vi "CloseFile.vi"(7 "Independent?":bool, 8 "error in (no error)":errorcluster, 10 "notifier in":refnum<notifier>, 11 "Refnum in":refnum<k34>) -> (0 "error out":errorcluster, 1 "Notifier out":refnum<notifier>, 2 "Not a refnum out":refnum<k34>, 3 "File Close action out":enum16{"Prompt", "Keep", "Archive", "Trash"}(ring))   [LabVIEW 2018]
panel:
  # "warning this VI is cloned when opened to prevent notification isses when called simultaneously make sure to edit the VI opened from explorer."
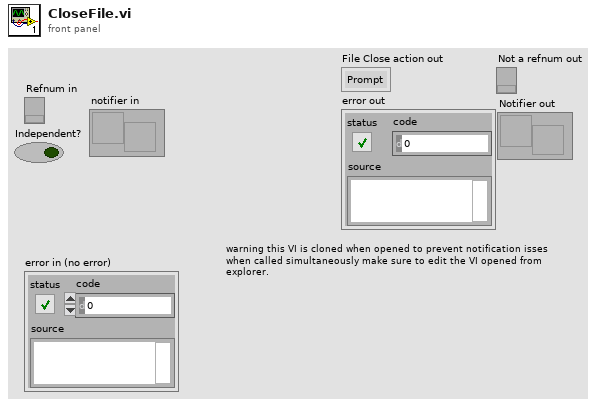
[diagram p1: front panel]
types:
  T1 = enum16{"Left Button", "Center Button", "Right Button", "Window Close"}
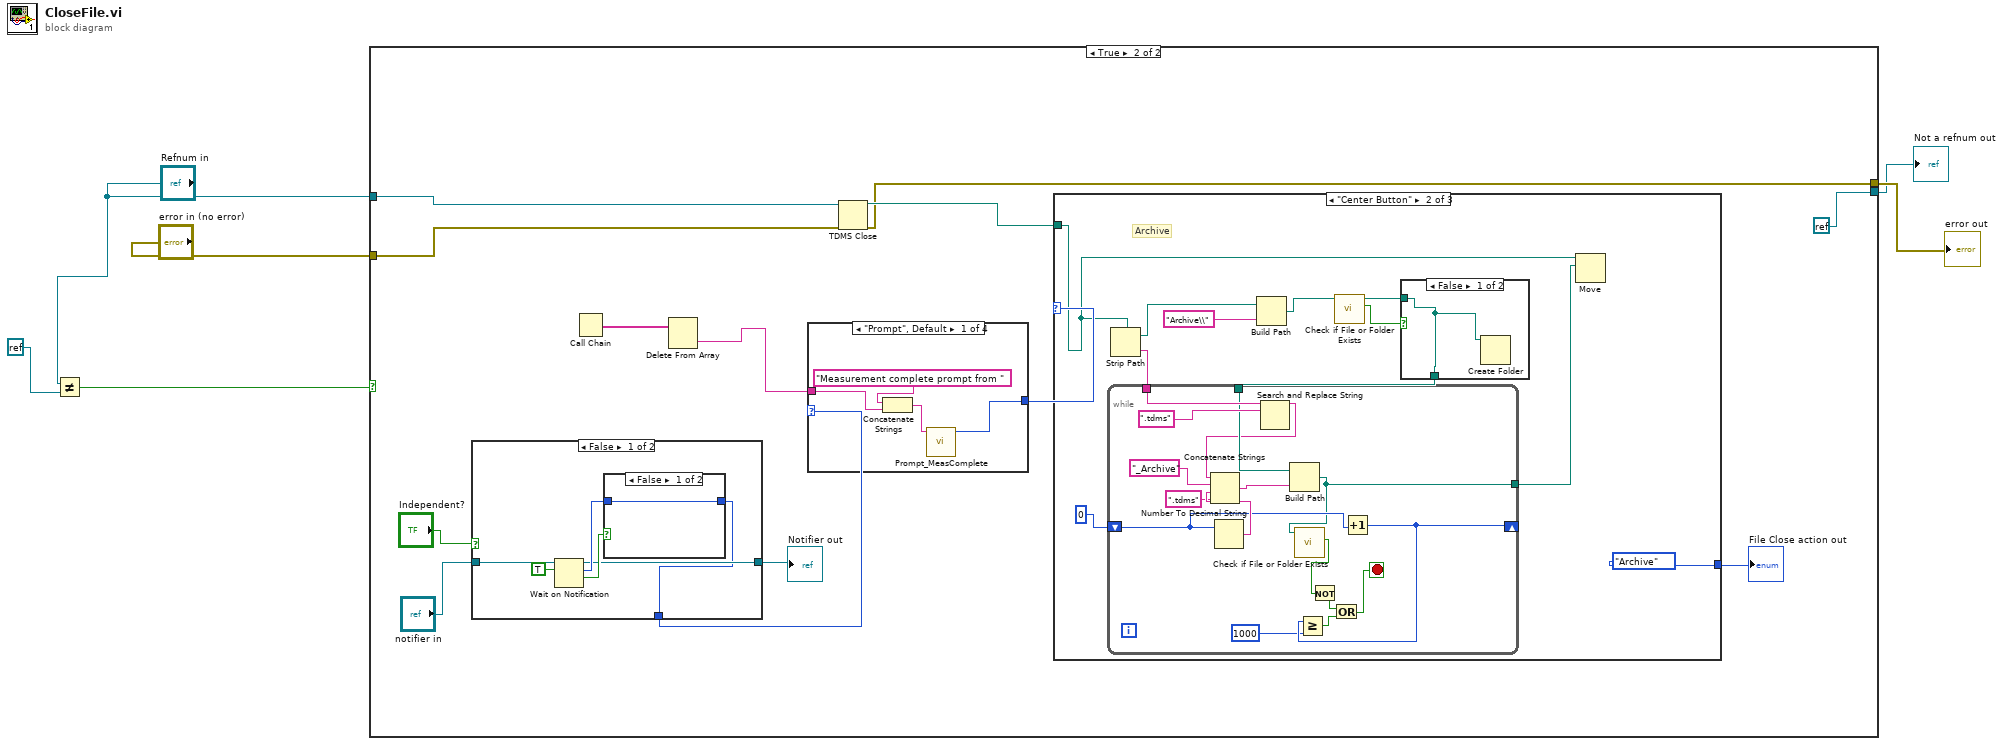
[diagram p0: block diagram]
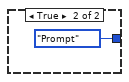
[diagram p3: hidden frame]
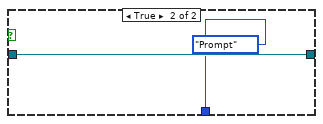
[diagram p4: hidden frame]
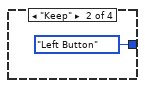
[diagram p5: hidden frame]
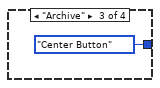
[diagram p6: hidden frame]
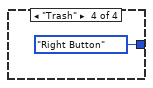
[diagram p7: hidden frame]
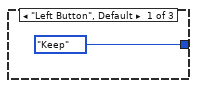
[diagram p8: hidden frame]
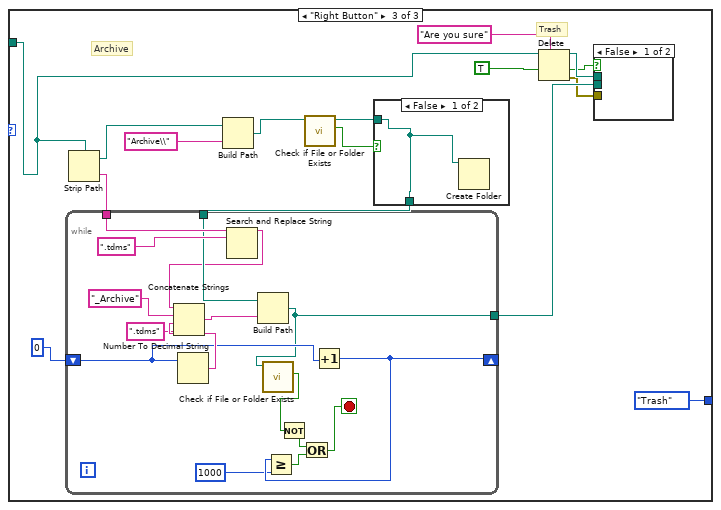
[diagram p10: hidden frame]
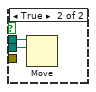
[diagram p11: hidden frame]
diagram:
  n1 = Not Equal?(x="Refnum in", y=refnum<k0> refnum) -> (x != y?=w3:bool)
  n2 = case shown="True" w3 {
    tunnel: "error in (no error)" -> [w7 w20]
    tunnel: "Refnum in" -> [w8 w18]
    tunnel: [w8 refnum<k0> refnum] -> w1
    tunnel: [w7 w16] -> w2
    frame False {
    }
    frame True {
      n3 = case shown="False" "Independent?" {
        tunnel: "notifier in" -> [w27 w31]
        tunnel: [w24 w31] -> w14
        tunnel: [w23 enum16{"Prompt", "Keep", "Archive", "Trash"}."Prompt" ("Action")] -> w11
        frame False {
          n4 = Wait on Notification(notifier=w27, ignore previous (F)=TRUE) -> (notifier out=w24:refnum<notifier>, notification=w25:enum16{"Prompt", "Keep", "Archive", "Trash"}, timed out?=w26:bool)  [unwired: 2 in, 1 out]
          n5 = case shown="False" w26 {
            tunnel: w25 -> [w28 _]
            tunnel: [w28 enum16{"Prompt", "Keep", "Archive", "Trash"}."Prompt" ("Action")] -> w23
            frame False {
            }
            frame True {
            }
          }
        }
        frame True {
        }
      }
      "Notifier out" <- w14
      n6 = Call Chain() -> (call chain=w10:string[])
      n7 = Delete From Array "Delete From Array"(array=w10) -> (deleted portion=w9:string)  [unwired: 2 in, 1 out]
      n8 = case shown="\"Prompt\", Default" w11 {
        tunnel: [w35 T1."Left Button" ("Which Button?") T1."Center Button" ("Which Button?") T1."Right Button" ("Which Button?")] -> w19
        tunnel: w9 -> [w34 _ _ _]
        frame "Prompt", Default {
          n9 = Concatenate Strings("Measurement complete prompt from " ("message"), w34) -> (w32:string)
          n10 = call "Prompt_MeasComplete.vi"("message"=w32) -> ("Which Button?"=w35:T1)  [unwired: 10 in]
        }
        frame "Keep" {
        }
        frame "Archive" {
        }
        frame "Trash" {
        }
      }
      n11 = TDMS Close(8:w20, 11:w18) -> (0:w16:errorcluster, 3:w21:path)
      n12 = case shown="\"Center Button\"" w19 {
        tunnel: w21 -> [_ w40 w72]
        tunnel: [enum16{"Prompt", "Keep", "Archive", "Trash"}."Keep" ("File Close action out") enum16{"Prompt", "Keep", "Archive", "Trash"}."Archive" ("File Close action out") enum16{"Prompt", "Keep", "Archive", "Trash"}."Trash" ("File Close action out")] -> w17
        frame "Left Button", Default {
        }
        frame "Center Button" {
          # "Archive"
          n13 = Strip Path(path=w40) -> (stripped path=w50:path, name=w48:string)
          n14 = Build Path(base path=w50, name or relative path="Archive\\") -> (appended path=w45:path)
          n15 = call <vilib>:"Check if File or Folder Exists.vi"("path"=w45) -> ("file or folder exists?"=w44:bool, "dup path"=w43:path)  [unwired: 8 in, 1 out]
          n16 = case shown="False" w44 {
            tunnel: w43 -> [w51 w52]
            tunnel: [w51 w52] -> w42
            frame False {
              n17 = Create Folder(path (use dialog)=w51) -> ()  [unwired: 2 in, 3 out]
            }
            frame True {
            }
          }
          n18 = while {
            tunnel: w48 -> [w68]
            tunnel: w42 -> [w66]
            shift-right: [w54] -> _
            shift-left: 0 -> [w60]
            tunnel: [w56] -> w46
            stop <- w57 stop-if-true
            n19 = Number To Decimal String(number=w60) -> (decimal integer string=w64:string)  [unwired: 1 in]
            n20 = Search and Replace String(input string=w68, search string=".tdms") -> (result string=w55:string)  [unwired: 6 in, 3 out]
            n21 = Concatenate Strings(w55, "_Archive" ("replace string (\"\")"), w64, ".tdms" ("string")) -> (w62:string)
            n22 = Build Path(base path=w66, name or relative path=w62) -> (appended path=w56:path)
            n23 = call <vilib>:"Check if File or Folder Exists.vi"("path"=w56) -> ("file or folder exists?"=w61:bool)  [unwired: 8 in, 2 out]
            n24 = Not(x=w61) -> (.not. x?=w59:bool)
            n25 = Increment(x=w60) -> (x+1=w54:i32)
            n26 = Greater Or Equal?(x=w54, y=1000) -> (x >= y?=w58:bool)
            n27 = Or(x=w59, y=w58) -> (x .or. y?=w57:bool)
          }
          n28 = Move(source path=w40, 10:w46) -> ()  [unwired: 3 in, 3 out]
        }
        frame "Right Button" {
          # "Trash"
          # "Archive"
          n29 = Strip Path(path=w72) -> (stripped path=w84:path, name=w82:string)
          n30 = Build Path(base path=w84, name or relative path="Archive\\") -> (appended path=w79:path)
          n31 = call <vilib>:"Check if File or Folder Exists.vi"("path"=w79) -> ("file or folder exists?"=w78:bool, "dup path"=w77:path)  [unwired: 8 in, 1 out]
          n32 = case shown="False" w78 {
            tunnel: w77 -> [w87 w88]
            tunnel: [w87 w88] -> w76
            frame False {
              n33 = Create Folder(path (use dialog)=w87) -> ()  [unwired: 2 in, 3 out]
            }
            frame True {
            }
          }
          n34 = while {
            tunnel: w82 -> [w104]
            tunnel: w76 -> [w102]
            shift-right: [w90] -> _
            shift-left: 0 -> [w96]
            tunnel: [w92] -> w80
            stop <- w93 stop-if-true
            n35 = Number To Decimal String(number=w96) -> (decimal integer string=w100:string)  [unwired: 1 in]
            n36 = Search and Replace String(input string=w104, search string=".tdms") -> (result string=w91:string)  [unwired: 6 in, 3 out]
            n37 = Concatenate Strings(w91, "_Archive" ("replace string (\"\")"), w100, ".tdms" ("string")) -> (w98:string)
            n38 = Build Path(base path=w102, name or relative path=w98) -> (appended path=w92:path)
            n39 = call <vilib>:"Check if File or Folder Exists.vi"("path"=w92) -> ("file or folder exists?"=w97:bool)  [unwired: 8 in, 2 out]
            n40 = Not(x=w97) -> (.not. x?=w95:bool)
            n41 = Increment(x=w96) -> (x+1=w90:i32)
            n42 = Greater Or Equal?(x=w90, y=1000) -> (x >= y?=w94:bool)
            n43 = Or(x=w95, y=w94) -> (x .or. y?=w93:bool)
          }
          n44 = Delete(prompt (Delete)="Are you sure", path (use dialog)=w72, confirm (F)=TRUE) -> (deleted path=w71:path, cancelled=w70:bool, error out=w69:errorcluster)  [unwired: 2 in]
          n45 = case shown="False" w70 {
            tunnel: w80 -> [_ w86]
            tunnel: w71 -> [_ w85]
            tunnel: w69 -> [_ _]
            frame False {
            }
            frame True {
              n46 = Move(source path=w85, 10:w86) -> ()  [unwired: 3 in, 3 out]
            }
          }
        }
      }
      "File Close action out" <- w17
    }
  }
  "error out" <- w2
  "Not a refnum out" <- w1
